vi "Scenario Add.vi"(8 "error in (no error)":errorcluster, 10 "Scenario Record":T1, 11 "Connection Refnum":T4) -> (0 "error out":errorcluster, 2 "New Scenario":T1, 3 "Connection Refnum":T4)   [LabVIEW 2011]
uses:
  Scenario Record.ctl
  Conditions/Condition Record.ctl
  Conditions/Condition Operators.ctl
  Summitek EXT/ODBC/SQL Controls/Connection Refnum.ctl
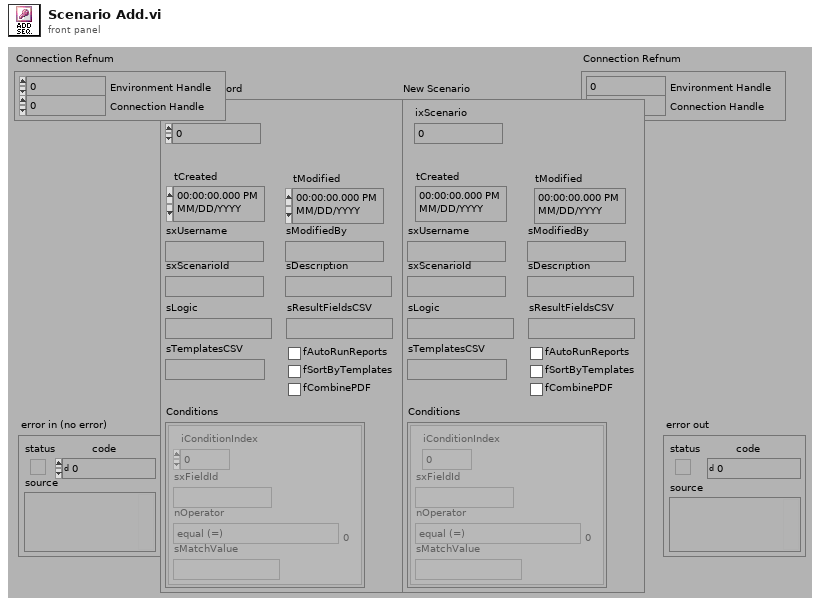
[diagram p1: front panel]
types:
  T1 = typedef "Scenario Record.ctl" = cluster{"ixScenario":i32, "tCreated":timestamp, "tModified":timestamp, "sxUsername":string, "sModifiedBy":string, "sxScenarioId":string, "sDescription":string, "sLogic":string, "sResultFieldsCSV":string, "sTemplatesCSV":string, "fAutoRunReports":bool, "fSortByTemplates":bool, "fCombinePDF":bool, "Conditions":T2[]}
  T2 = typedef "Condition Record.ctl" = cluster{"iConditionIndex":i32, "sxFieldId":string, "nOperator":T3, "sMatchValue":string}
  T3 = typedef "Condition Operators.ctl" = enum16{"equal (=)", "not equal (\\u2260)", "less than (<)", "less than or equal (\\u2264)", "greater than (>)", "greater than or equal (\\u2265)", "contains", "does not contain"}
  T4 = typedef "Connection Refnum.ctl" = cluster{"Environment Handle":i32, "Connection Handle":i32}
  T5 = typedef "Statement Refnum.ctl" = cluster{"Statement Handle":i32, "Parameter Number":u16}
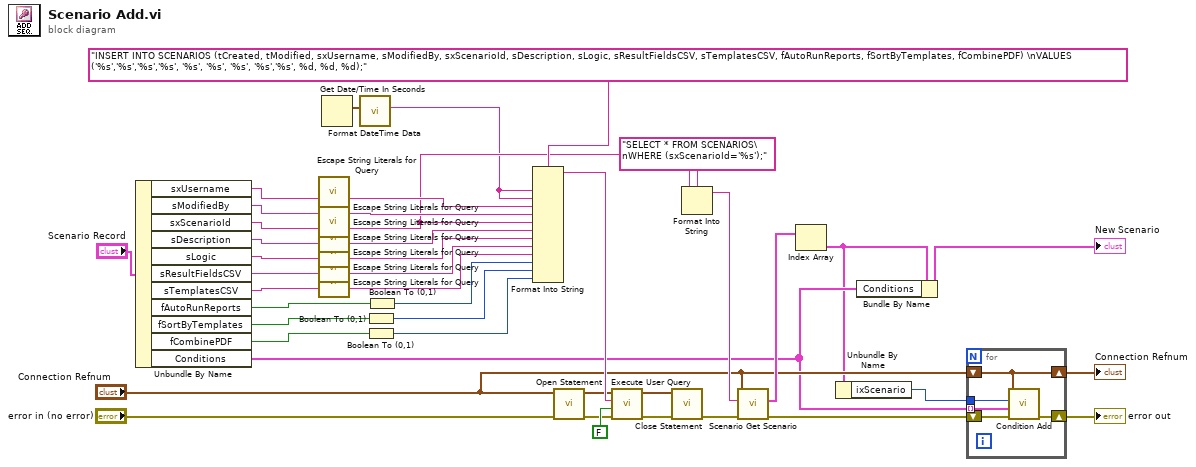
[diagram p0: block diagram]
diagram:
  n1 = Unbundle By Name("Scenario Record") -> ("sxUsername"=w35:string, "sModifiedBy"=w27:string, "sxScenarioId"=w34:string, "sDescription"=w33:string, "sLogic"=w24:string, "sResultFieldsCSV"=w22:string, "sTemplatesCSV"=w9:string, "fAutoRunReports"=w2:bool, "fSortByTemplates"=w7:bool, "fCombinePDF"=w5:bool, "Conditions"=w13:T2[])
  n2 = call "Escape String Literals for Query.vi"("String"=w35) -> ("escaped String"=w28:string)  [unwired: 1 in, 13 out]
  n3 = call "Escape String Literals for Query.vi"("String"=w27) -> ("escaped String"=w26:string)  [unwired: 1 in, 13 out]
  n4 = call "Escape String Literals for Query.vi"("String"=w34) -> ("escaped String"=w20:string)  [unwired: 1 in, 13 out]
  n5 = call "Escape String Literals for Query.vi"("String"=w33) -> ("escaped String"=w25:string)  [unwired: 1 in, 13 out]
  n6 = call "Escape String Literals for Query.vi"("String"=w24) -> ("escaped String"=w23:string)  [unwired: 1 in, 13 out]
  n7 = call "Escape String Literals for Query.vi"("String"=w22) -> ("escaped String"=w21:string)  [unwired: 1 in, 13 out]
  n8 = call "Escape String Literals for Query.vi"("String"=w9) -> ("escaped String"=w10:string)  [unwired: 1 in, 13 out]
  n9 = Get Date/Time In Seconds() -> (seconds since 1Jan1904=w8:timestamp)
  n10 = call "Format DateTime Data.vi"("Timestamp in"=w8) -> ("UTC DB String out"=w3:string)  [unwired: 10 out]
  n11 = Boolean To (0,1)(Boolean=w7) -> (0, 1=w6:i16)
  n12 = Boolean To (0,1)(Boolean=w5) -> (0, 1=w4:i16)
  n13 = Boolean To (0,1)(Boolean=w2) -> (0, 1=w1:i16)
  n14 = Format Into String(format string="INSERT INTO SCENARIOS (tCreated, tModified, sxUsername, sModifiedBy, sxScenarioId, sDescription, sLogic, sResultFieldsCSV, sTemplatesCSV, fAutoRunReports, fSortByTemplates, fCombinePDF) \nVALUES ('%s','%s','%s','%s', '%s', '%s', '%s', '%s','%s', %d, %d, %d);" ("User Query"), w3, w3, w28, w26, w20, w25, w23, w21, w10, w1, w6, w4) -> (resulting string=w41:string)  [unwired: 2 in, 1 out]
  n15 = call "Open Statement.vi"("error in (no error)"="error in (no error)", "Connection Refnum"="Connection Refnum") -> ("error out"=w37:errorcluster, "Statement Refnum"=w36:T5)  [unwired: 4 out]
  n16 = call "Execute User Query.vi"("error in (no error)"=w37, "Return Data? (f)"=FALSE, "User Query"=w41, "Statement Refnum"=w36) -> ("error out"=w38:errorcluster, "Statement Refnum"=w39:T5)  [unwired: 2 out]
  n17 = call "Close Statement.vi"("error in (no error)"=w38, "Statement Refnum"=w39) -> ("error out"=w19:errorcluster)  [unwired: 5 out]
  n18 = Format Into String(format string="SELECT * FROM SCENARIOS\nWHERE (sxScenarioId='%s');", w20) -> (resulting string=w29:string)  [unwired: 2 in, 1 out]
  n19 = call "Scenario Get Scenario.vi"("error in (no error)"=w19, "Query"=w29, "Connection Refnum"="Connection Refnum") -> ("error out"=w17:errorcluster, "Scenarios"=w31:T1[])  [unwired: 7 out]
  n20 = Index Array(array=w31) -> (element=w12:T1)  [unwired: 1 in]
  n21 = Unbundle By Name(w12) -> ("ixScenario"=w11:i32)
  n22 = Bundle By Name(cluster=w12, "Conditions"=w13) -> (→"New Scenario":T1)
  n23 = for {
    shift-right: [w46] -> w18
    shift-left: "Connection Refnum" -> [w46]
    shift-right: [w47] -> w16
    shift-left: w17 -> [w48]
    tunnel: w13 -> [w45] mode=indexing
    tunnel: w11 -> [w44]
    n24 = call "Condition Add.vi"("error in (no error)"=w48, "Condition"=w45, "ixScenario (0)"=w44, "Connection Refnum"=w46) -> ("error out"=w47:errorcluster)  [unwired: 7 out]
  }
  "error out" <- w16
  "Connection Refnum" <- w18
